vi "Launch Async File Reader.vi"(8 "error in (no error)":errorcluster, 9 "Command FIFO":refnum<k33>, 10 "New Values FIFO":refnum<k33>, 11 "Device Reference in":T1 format="%.0x") -> (0 "error out":errorcluster, 3 "Device Reference Out":T1 format="%.0x")   [LabVIEW 2011, in "Interpolate 1D Array Custom Device.lvlib"]
doc: "Launches a VI which waits on the 'Command FIFO' and then re-reads the spreadsheet and brings the new data back via the 'New Values FIFO'."
uses:
  Interpolate 1D Array Custom Device.lvlib
  <vilib>/NI Veristand/Custom Device API/Custom Device Item Ref.ctl
  Async File Reader.vi
  <vilib>/NI Veristand/Custom Device API/Custom Device API.lvlib
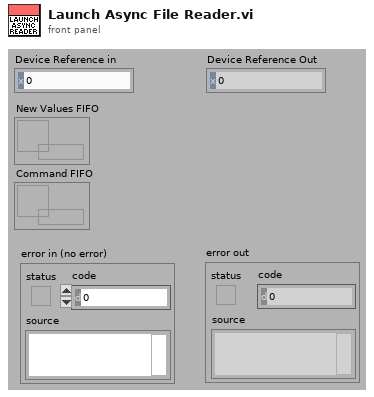
[diagram p1: front panel]
types:
  T1 = typedef "Custom Device API.lvlib/Custom Device Item Ref.ctl" = u64
  T2 = cluster{"Device Reference in":T1, "New Values FIFO":refnum<k33>, "Command FIFO":refnum<k33>}
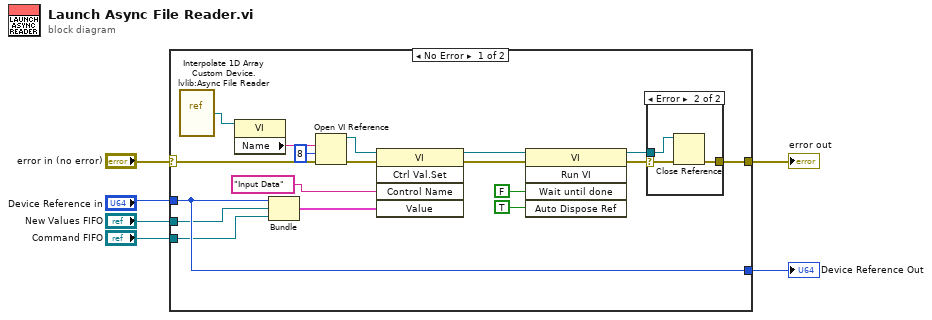
[diagram p0: block diagram]
diagram:
  n1 = case shown="No Error" "error in (no error)" {
    selector: "error in (no error)" -> [w22 w30]
    tunnel: [w18 w30] -> w6
    tunnel: "Device Reference in" -> [w13 w29]
    tunnel: "New Values FIFO" -> [w12 _]
    tunnel: "Command FIFO" -> [w11 _]
    tunnel: [w13 w29] -> w1
    frame No Error {
      n2 = vi-ref "Interpolate 1D Array Custom Device.lvlib:Async File Reader.vi"() -> (w16:refnum<vi>)
      n3 = property class="VI"(reference=w16) -> ("Name"=w24:string)  [unwired: 1 in, 2 out]
      n4 = Bundle("Device Reference in"=w13, "New Values FIFO"=w12, "Command FIFO"=w11) -> (w7:T2)  [unwired: 1 out]
      n5 = Open VI Reference(vi path=w24, options=8, error in (no error)=w22) -> (vi reference=w17:refnum<vi>, error out=w14:errorcluster)  [unwired: 3 out]
      n6 = invoke class="VI" method="Ctrl Val.Set"(reference=w17, error in=w14, "Control Name"="Input Data", "Value"=w7) -> (reference out=w10:refnum<vi>, error out=w9:errorcluster)  [unwired: 1 in, 3 out]
      n7 = invoke class="VI" method="Run VI"(reference=w10, error in=w9, "Wait until done"=FALSE ("Wait Until Done"), "Auto Dispose Ref"=TRUE ("Auto Dispose Reference")) -> (reference out=w19:refnum<vi>, error out=w15:errorcluster)  [unwired: 1 in, 3 out]
      n8 = case shown="Error" w15 {
        selector: w15 -> [w25 w28]
        tunnel: w19 -> [_ w27]
        tunnel: [w25 w26] -> w18
        frame No Error {
        }
        frame Error {
          n9 = Close Reference(reference=w27, error in (no error)=w28) -> (error out=w26:errorcluster)
        }
      }
    }
    frame Error {
    }
  }
  "error out" <- w6
  "Device Reference Out" <- w1
